vi "Write hostLoopPeriod_s.vi"(8 "error in (no error)":errorcluster, 10 "hostLoopPeriod_s":dbl=0.016, 11 "LoopConfig in":refnum<class "LoopConfig.lvclass">) -> (0 "error out":errorcluster, 3 "LoopConfig out":refnum<class "LoopConfig.lvclass">)   [LabVIEW 2013, in "ComponentData.lvlib" / "LoopConfig.lvclass"]
uses:
  <userlib>/Common/Component/common_application/RT/ComponentData/ConfigurationHandler/LoopConfig/LoopConfig.lvclass
  <userlib>/Common/Component/common_application/RT/ComponentData/ConfigurationHandler/LoopConfig/LoopConfig.lvclass/LoopConfig.ctl
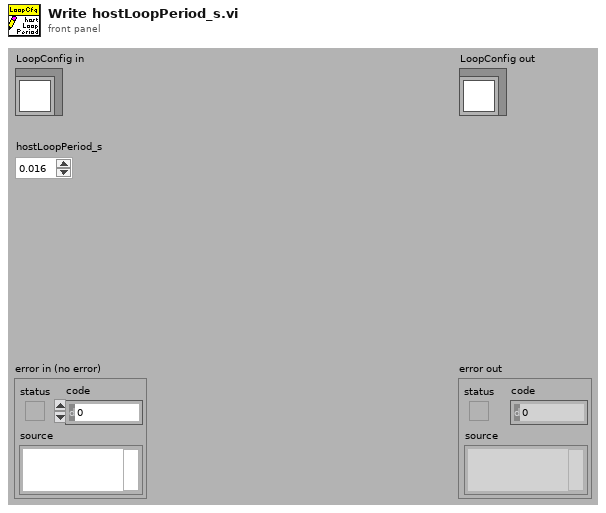
[diagram p1: front panel]
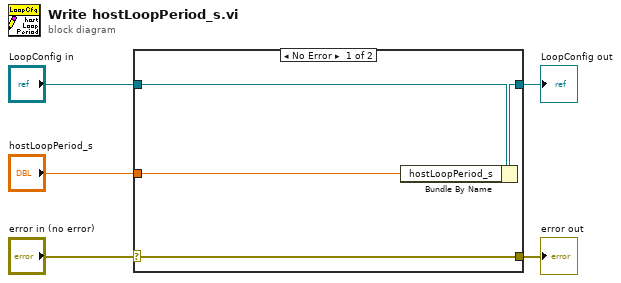
[diagram p0: block diagram]
diagram:
  n1 = case shown="No Error" "error in (no error)" {
    selector: "error in (no error)" -> [w9 w10]
    tunnel: [w9 w10] -> w4
    tunnel: [w7 w11] -> w2
    tunnel: "LoopConfig in" -> [w8 w11]
    tunnel: "hostLoopPeriod_s" -> [w6 _]
    frame No Error {
      n2 = Bundle By Name(cluster=w8, "hostLoopPeriod_s"=w6) -> (w7:refnum<class "LoopConfig.lvclass">)
    }
    frame Error {
    }
  }
  "error out" <- w4
  "LoopConfig out" <- w2
